vi "calculation.vi"(0 "Counter\nInput":dbl) -> (1 "Counter\nOutput":dbl, 2 "Temperature\nOutput":dbl)   [LabVIEW 2023]
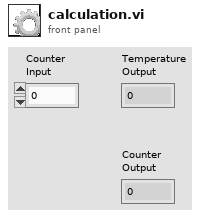
[diagram p1: front panel]
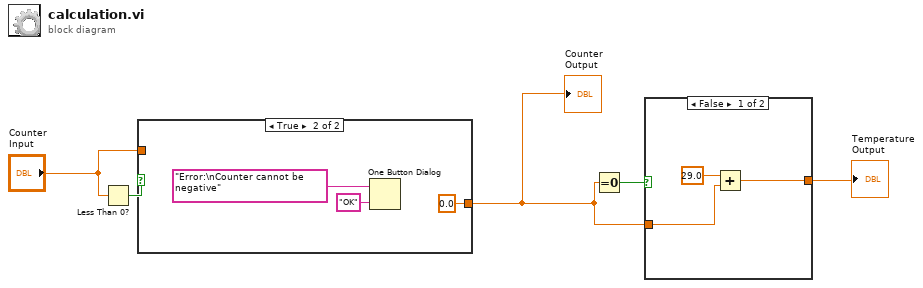
[diagram p0: block diagram]
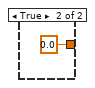
[diagram p2: hidden frame]
diagram:
  n1 = Less Than 0?(x="Counter\nInput") -> (x < 0?=w3:bool)
  n2 = case shown="True" w3 {
    tunnel: [w6 0.0] -> w1
    tunnel: "Counter\nInput" -> [w6 _]
    frame False {
    }
    frame True {
      n3 = One Button Dialog(message="Error:\nCounter cannot be negative" ("error source (\" \")"), button name ("OK")="OK") -> ()  [unwired: 1 out]
    }
  }
  "Counter\nOutput" <- w1
  n4 = Equal To 0?(x=w1) -> (x = 0?=w4:bool)
  n5 = case shown="False" w4 {
    tunnel: w1 -> [w11 _]
    tunnel: [w10 0.0] -> w5
    frame False {
      n6 = Add(x=29.0, y=w11) -> (x+y=w10:dbl)
    }
    frame True {
    }
  }
  "Temperature\nOutput" <- w5
